vi "CODMn手动控制框.vi"(8 "Error in":errorcluster) -> ()   [LabVIEW 2016, in "斯坦道CODMn.lvlib"]
uses:
  <vilib>/Plasmionique/MB Master/MB Master.lvlib
panel:
  in  "草酸钠":bool
  in  "高锰酸钾":bool
  in  "常规版/认证版":enum16{"常规版", "认证版"}(ring)
  in  "高锰酸钾滴定（10uL每滴）":bool
  in  "草酸钠泵排":bool
  in  "草酸钠泵进":bool
  in  "草酸钠泵复位":bool
  in  "高锰酸钾泵排":bool
  in  "高锰酸钾泵进":bool
  in  "高锰酸钾泵复位":bool
  in  "风扇":bool
  in  "排液":bool
  in  "搅拌":bool
  in  "加热":bool
  in  "硫酸":bool
  in  "加标回收样":bool
  in  "质控样":bool
  in  "标液":bool
  in  "纯水":bool
  in  "退出":bool
  in  "水样":bool
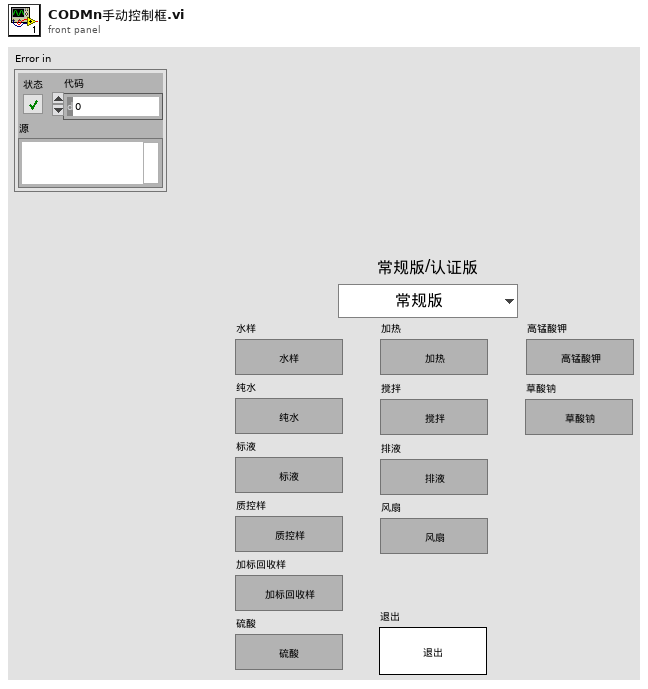
[diagram p1: front panel]
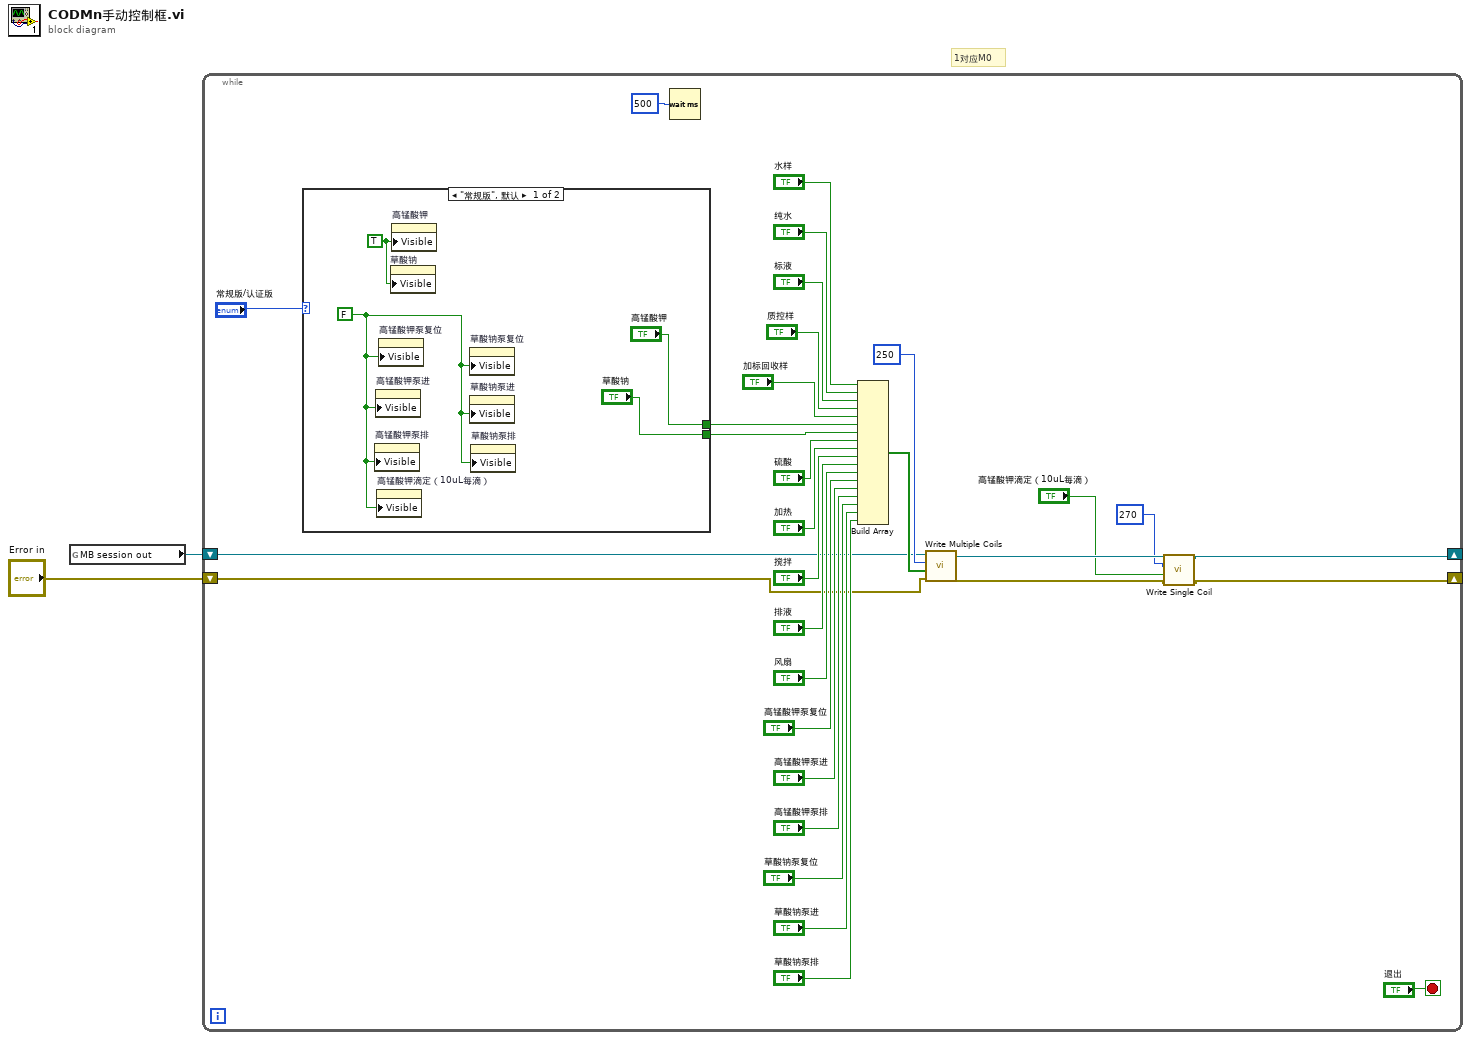
[diagram p0: block diagram]
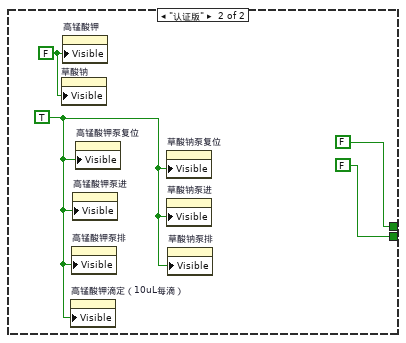
[diagram p2: hidden frame]
diagram:
  # "1对应M0"
  n1 = global read "CODMn断电保存全局变量.vi" "MB session out"() -> (w1:refnum<class "MB_Master.lvclass">)
  n2 = while {
    shift-right: [w7] -> _
    shift-left: w1 -> [w13]
    shift-right: [w6] -> _
    shift-left: "Error in" -> [w12]
    stop <- "退出" stop-if-true
    n3 = case shown="\"常规版\", 默认" "常规版/认证版" {
      tunnel: ["高锰酸钾" FALSE ("元素")] -> w4
      tunnel: ["草酸钠" FALSE ("元素")] -> w3
      frame "常规版", Default {
        w36 = FALSE ("可见")
        w37 = TRUE ("可见")
        n4 = property on="高锰酸钾泵排" class="Bool (严格)"("Visible"=w36) -> ()  [unwired: 2 in, 2 out]
        n5 = property on="高锰酸钾泵进" class="Bool (严格)"("Visible"=w36) -> ()  [unwired: 2 in, 2 out]
        n6 = property on="高锰酸钾滴定（10uL每滴）" class="Bool (严格)"("Visible"=w36) -> ()  [unwired: 2 in, 2 out]
        n7 = property on="高锰酸钾泵复位" class="Bool (严格)"("Visible"=w36) -> ()  [unwired: 2 in, 2 out]
        n8 = property on="草酸钠" class="Bool (严格)"("Visible"=w37) -> ()  [unwired: 2 in, 2 out]
        n9 = property on="高锰酸钾" class="Bool (严格)"("Visible"=w37) -> ()  [unwired: 2 in, 2 out]
        n10 = property on="草酸钠泵复位" class="Bool (严格)"("Visible"=w36) -> ()  [unwired: 2 in, 2 out]
        n11 = property on="草酸钠泵进" class="Bool (严格)"("Visible"=w36) -> ()  [unwired: 2 in, 2 out]
        n12 = property on="草酸钠泵排" class="Bool (严格)"("Visible"=w36) -> ()  [unwired: 2 in, 2 out]
      }
      frame "认证版" {
        w40 = TRUE ("可见")
        w41 = FALSE ("可见")
        n13 = property on="草酸钠" class="Bool (严格)"("Visible"=w41) -> ()  [unwired: 2 in, 2 out]
        n14 = property on="高锰酸钾" class="Bool (严格)"("Visible"=w41) -> ()  [unwired: 2 in, 2 out]
        n15 = property on="高锰酸钾滴定（10uL每滴）" class="Bool (严格)"("Visible"=w40) -> ()  [unwired: 2 in, 2 out]
        n16 = property on="高锰酸钾泵排" class="Bool (严格)"("Visible"=w40) -> ()  [unwired: 2 in, 2 out]
        n17 = property on="高锰酸钾泵进" class="Bool (严格)"("Visible"=w40) -> ()  [unwired: 2 in, 2 out]
        n18 = property on="高锰酸钾泵复位" class="Bool (严格)"("Visible"=w40) -> ()  [unwired: 2 in, 2 out]
        n19 = property on="草酸钠泵复位" class="Bool (严格)"("Visible"=w40) -> ()  [unwired: 2 in, 2 out]
        n20 = property on="草酸钠泵进" class="Bool (严格)"("Visible"=w40) -> ()  [unwired: 2 in, 2 out]
        n21 = property on="草酸钠泵排" class="Bool (严格)"("Visible"=w40) -> ()  [unwired: 2 in, 2 out]
      }
    }
    n22 = Wait (ms)(milliseconds to wait=u32 500 ("等待时间（毫秒）")) -> ()  [unwired: 1 out]
    n23 = Build Array("水样", "纯水", "标液", "质控样", "加标回收样", w4, w3, "硫酸", "加热", "搅拌", "排液", "风扇", "高锰酸钾泵复位", "高锰酸钾泵进", "高锰酸钾泵排", "草酸钠泵复位", "草酸钠泵进", "草酸钠泵排") -> (w30:bool[])
    n24 = call <vilib>:"Write Multiple Coils.vi"("error in (no error)"=w12, "values"=w30, "starting address"=u16 250, "MB session in"=w13) -> ("error out"=w9:errorcluster, "MB session out"=w11:refnum<class "MB_Master.lvclass">)  [unwired: 6 in]
    n25 = call <vilib>:"Write Single Coil.vi"("error in (no error)"=w9, "value"="高锰酸钾滴定（10uL每滴）", "address"=u16 270 ("starting address"), "MB session in"=w11) -> ("error out"=w6:errorcluster, "MB session out"=w7:refnum<class "MB_Master.lvclass">)  [unwired: 6 in]
  }
